vi "Read Write Unicode File _APTLib.vi"(6 "Option":T2, 8 "error in":errorcluster, 9 "Encoding?":T1=enum."UTF-8", 10 "String In":string, 11 "file path":path) -> (0 "error out":errorcluster, 2 "String Out":string, 3 "file path Out":path)   [LabVIEW 2019]
uses:
  <userlib>/APTLib.lnk/File IO/_Read Write Data File _APTLib.llb/File IO Option _APTLib.ctl
  <userlib>/APTLib.lnk/File IO/_Read Write Data File _APTLib.llb/Text Encoding Format _APTLib.ctl
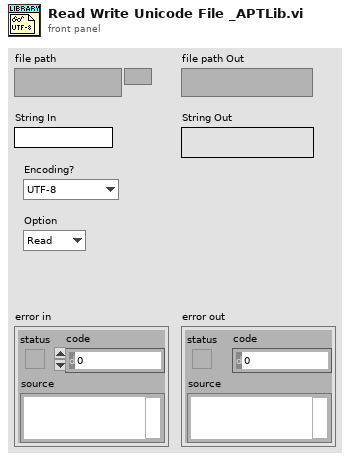
[diagram p1: front panel]
types:
  T1 = typedef "Text Encoding Format _APTLib.ctl" = enum8{"ASCII", "UTF-8", "UTF-16 LE", "UTF-16 BE"}
  T2 = typedef "File IO Option _APTLib.ctl" = enum16{"Read", "Write"}
  T3 = enum16{"open", "replace", "create", "open or create", "replace or create", "replace or create with confirmation"}
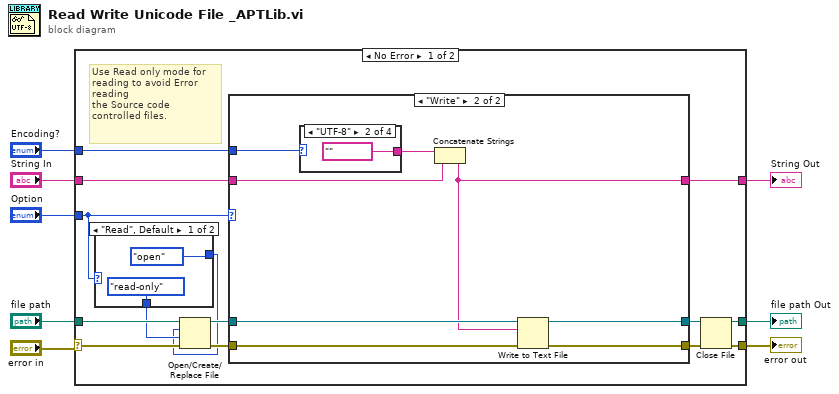
[diagram p0: block diagram]
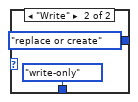
[diagram p2: hidden frame]
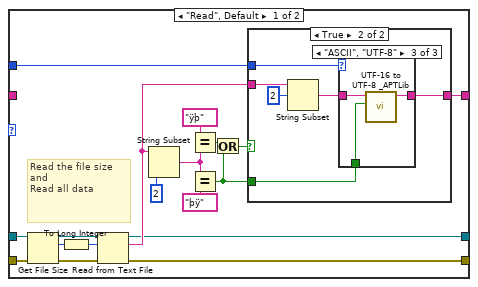
[diagram p3: hidden frame]
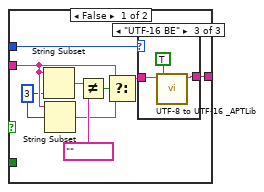
[diagram p4: hidden frame]
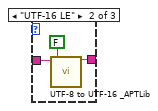
[diagram p6: hidden frame]
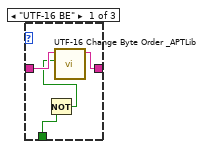
[diagram p7: hidden frame]
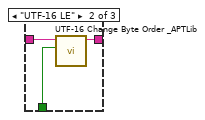
[diagram p8: hidden frame]
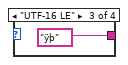
[diagram p10: hidden frame]
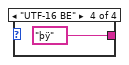
[diagram p11: hidden frame]
diagram:
  n1 = case shown="No Error" "error in" {
    selector: "error in" -> [w19 w90]
    tunnel: [w21 w90] -> w6
    tunnel: "file path" -> [w20 w89]
    tunnel: [w22 w88] -> w2
    tunnel: [w13 w89] -> w7
    tunnel: "String In" -> [w12 w88]
    tunnel: "Option" -> [w11 _]
    tunnel: "Encoding?" -> [w10 _]
    frame No Error {
      # "Use Read only mode for \nreading to avoid Error reading \nthe Source code controlled files."
      n2 = case shown="\"Read\", Default" w11 {
        tunnel: [enum16{"read/write", "read-only", "write-only"}."read-only" ("access (0:read/write)") enum16{"read/write", "read-only", "write-only"}."write-only" ("access (0:read/write)")] -> w16
        tunnel: [T3."open" ("operation (0:open)") T3."replace or create" ("operation (0:open)")] -> w9
        frame "Read", Default {
        }
        frame "Write" {
        }
      }
      n3 = Open/Create/Replace File(file path (use dialog)=w20, error in=w19, operation (0:open)=w9, access (0:read/write)=w16) -> (refnum out=w15:refnum<file>, error out=w14:errorcluster)  [unwired: 2 in, 1 out]
      n4 = case shown="\"Write\"" w11 {
        tunnel: [w37 w77] -> w22
        tunnel: [w35 w82] -> w18
        tunnel: [w34 w81] -> w17
        tunnel: w15 -> [w32 w84]
        tunnel: w14 -> [w30 w83]
        tunnel: w12 -> [_ w79]
        tunnel: w10 -> [w33 w80]
        frame "Read", Default {
          # "Read the file size and \nRead all data"
          n5 = Get File Size(file=w32, error in=w30) -> (refnum out=w31:refnum<file>, size (in bytes)=w28:i64, 0:w29:errorcluster)
          n6 = To Long Integer(number=w28) -> (32bit integer=w27:i32)
          n7 = Read from Text File(file (use dialog)=w31, count=w27, error in=w29) -> (refnum out=w35:refnum<file>, text=w36:string, error out=w34:errorcluster)  [unwired: 1 in, 1 out]
          n8 = String Subset(string=w36, length (rest)=2 ("length (rest)")) -> (substring=w42:string)  [unwired: 1 in]
          n9 = Equal?(x="ÿþ" ("text 2"), y=w42) -> (x = y?=w39:bool)
          n10 = Equal?(x=w42, y="þÿ" ("text 2")) -> (x = y?=w40:bool)
          n11 = Or(x=w39, y=w40) -> (x .or. y?=w38:bool)
          n12 = case shown="True" w38 {
            tunnel: w36 -> [w49 w65]
            tunnel: [w46 w64] -> w37
            tunnel: w40 -> [_ w62]
            tunnel: w33 -> [w47 w61]
            frame False {
              w48 = 3 ("offset (0)")
              n13 = String Subset(string=w49, length (rest)=w48) -> (substring=w52:string)  [unwired: 1 in]
              n14 = String Subset(string=w49, offset (0)=w48) -> (substring=w50:string)  [unwired: 1 out]
              n15 = Not Equal?(x=w52, y="﻿" ("text 2")) -> (x != y?=w51:bool)
              n16 = Select(t=w49, s=w51, f=w50) -> (s? t:f=w45:string)
              n17 = case shown="\"UTF-16 BE\"" w47 {
                tunnel: [w54 w55 w59] -> w46
                tunnel: w45 -> [w54 w57 w60]
                frame "ASCII", "UTF-8" {
                }
                frame "UTF-16 LE" {
                  n18 = call <userlib>:"UTF-8 to UTF-16 _APTLib.vi"("Big Endian?"=FALSE, "UTF-8 String"=w57) -> ("UTF-16 String"=w55:string)  [unwired: 8 in, 1 out]
                }
                frame "UTF-16 BE" {
                  n19 = call <userlib>:"UTF-8 to UTF-16 _APTLib.vi"("Big Endian?"=TRUE, "UTF-8 String"=w60) -> ("UTF-16 String"=w59:string)  [unwired: 8 in, 1 out]
                }
              }
            }
            frame True {
              n20 = String Subset(string=w65, offset (0)=2) -> (substring=w63:string)  [unwired: 1 out]
              n21 = case shown="\"ASCII\", \"UTF-8\"" w61 {
                tunnel: [w67 w71 w74] -> w64
                tunnel: w63 -> [w69 w73 w76]
                tunnel: w62 -> [w70 w72 w75]
                frame "UTF-16 BE" {
                  n22 = Not(x=w70) -> (.not. x?=w68:bool)
                  n23 = call <userlib>:"UTF-16 Change Byte Order _APTLib.vi"("Change BO?"=w68, "UTF-16 String In"=w69) -> ("UTF-16 String Out"=w67:string)  [unwired: 8 in, 1 out]
                }
                frame "UTF-16 LE" {
                  n24 = call <userlib>:"UTF-16 Change Byte Order _APTLib.vi"("Change BO?"=w72, "UTF-16 String In"=w73) -> ("UTF-16 String Out"=w71:string)  [unwired: 8 in, 1 out]
                }
                frame "ASCII", "UTF-8" {
                  n25 = call <userlib>:"UTF-16 to UTF-8 _APTLib.vi"("Big Endian?"=w75, "UTF-16 String"=w76) -> ("UTF-8 String"=w74:string)  [unwired: 8 in, 1 out]
                }
              }
            }
          }
        }
        frame "Write" {
          n26 = case shown="\"UTF-8\"" w80 {
            tunnel: [_ "﻿" ("text 2") "ÿþ" ("text 2") "þÿ" ("text 2")] -> w78
            frame "ASCII", Default {
            }
            frame "UTF-8" {
            }
            frame "UTF-16 LE" {
            }
            frame "UTF-16 BE" {
            }
          }
          n27 = Concatenate Strings(w78, w79) -> (w77:string)
          n28 = Write to Text File(file (use dialog)=w84, text=w77, error in=w83) -> (refnum out=w82:refnum<file>, error out=w81:errorcluster)  [unwired: 1 in, 1 out]
        }
      }
      n29 = Close File(refnum=w18, error in=w17) -> (path=w13:path, error out=w21:errorcluster)
    }
    frame Error {
      # "Upon Error Do Nothing"
    }
  }
  "String Out" <- w2
  "error out" <- w6
  "file path Out" <- w7
